vi "Insert Map of Created Attributes.vi"(10 "Created Attributes":refnum<class "Attributes.lvclass">, 11 "Base Actor in":refnum<class "Base Actor.lvclass">) -> (3 "Base Actor out":refnum<class "Base Actor.lvclass">)   [LabVIEW 2020, in "jettl.lvlib" / "Actor.lvlib" / "Base Actor.lvclass"]
uses:
  Base Actor.lvclass
  Attributes/Attributes/Attributes.lvclass
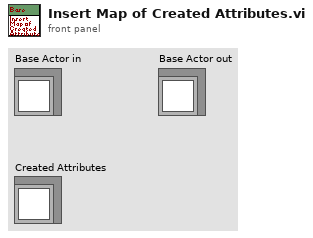
[diagram p1: front panel]
types:
  T1 = typedef "jettl.lvlib/Actor.lvlib/Map of Created Attributes.ctl" = map{string, refnum<class "Attributes.lvclass">}
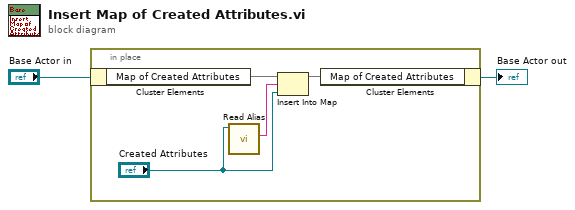
[diagram p0: block diagram]
diagram:
  n1 = in-place {
    n2 = in-place-cluster #1("Base Actor in") -> ("Map of Created Attributes"=w6:T1)
    n3 = call-dynamic "Read Alias.vi"("Attributes in"="Created Attributes") -> ("Alias"=w4:string)  [unwired: 10 in]
    n4 = Insert Into Map(map in=w6, key=w4, value="Created Attributes") -> (map out=w5:T1)  [unwired: 2 out]
    n5 = in-place-cluster #1("Map of Created Attributes"=w5) -> (→"Base Actor out":refnum<class "Base Actor.lvclass">)
  }
